vi "_Serial_buf clear.vi"(3 "에러 출력 2":errorcluster caption="에러 입력", 5 "Serial Port":refnum<visa-resource-name>="COM3") -> (0 "에러 출력":errorcluster, 2 "Serial Port 2":refnum<visa-resource-name>="COM3")   [LabVIEW 2015]
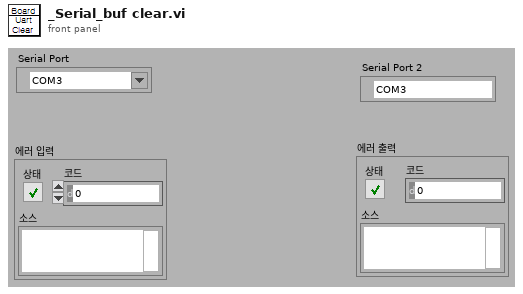
[diagram p1: front panel]
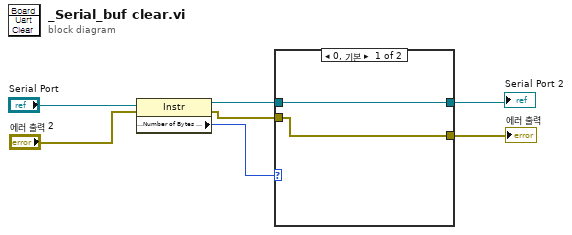
[diagram p0: block diagram]
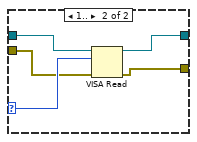
[diagram p2: hidden frame]
diagram:
  n1 = property class="Instr"(reference="Serial Port", error in="에러 출력 2") -> (reference out=w4:refnum<visa-resource-name>, error out=w2:errorcluster, "Serial Settings:Number of Bytes at Serial Port"=w5:u32)
  n2 = case shown="0, 기본" w5 {
    selector: w5 -> [_ w12]
    tunnel: w4 -> [w9 w14]
    tunnel: [w9 w13] -> w3
    tunnel: w2 -> [w8 w11]
    tunnel: [w8 w10] -> w1
    frame 0, Default {
    }
    frame 1.. {
      n3 = VISA Read(VISA resource name=w14, byte count=w12, error in (no error)=w11) -> (VISA resource name out=w13:refnum<visa-resource-name>, error out=w10:errorcluster)  [unwired: 2 out]
    }
  }
  "Serial Port 2" <- w3
  "에러 출력" <- w1
